vi "Set Read Timeout.vi"(10 "Read Timeout":i32=-1 format="%.0f ms", 11 "Reply Protocol Base in":refnum<class "Reply Protocol Base.lvclass">) -> (3 "Reply Protocol Base out":refnum<class "Reply Protocol Base.lvclass">)   [LabVIEW 2023, in "HAL GOOP4.lvlib" / "Reply Protocol Base.lvclass"]
uses:
  Reply Protocol Base.lvclass
  Reply Protocol Base.lvclass/Reply Protocol Base.ctl
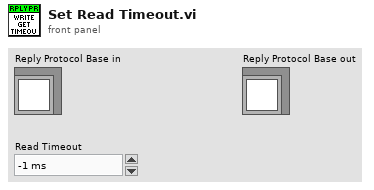
[diagram p1: front panel]
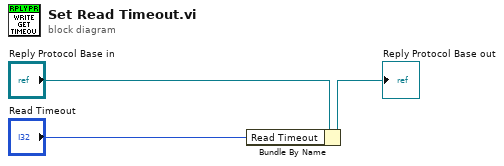
[diagram p0: block diagram]
diagram:
  n1 = Bundle By Name(cluster="Reply Protocol Base in", "Read Timeout"="Read Timeout") -> (→"Reply Protocol Base out":refnum<class "Reply Protocol Base.lvclass">)
